vi "Unmarshal.vi"(8 "error in (no error)":errorcluster, 10 "Buffer":u8[](array[numeric]), 11 "int32 in":refnum<class "double.lvclass">) -> (0 "error out":errorcluster, 2 "Buffer Count":i32=8, 3 "int32 out":refnum<class "double.lvclass">)   [LabVIEW 2020, in "Protobuf RAW.lvlib" / "double.lvclass"]
uses:
  double.lvclass
  double.lvclass/double.ctl
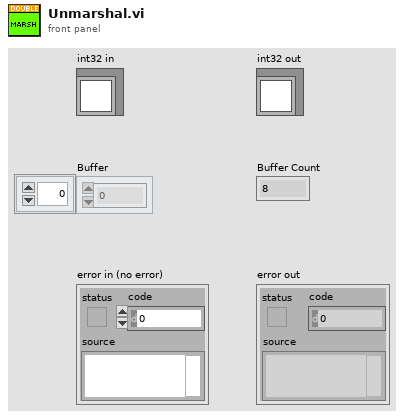
[diagram p1: front panel]
types:
  T1 = enum16{"big-endian, network order", "native, host order", "little-endian"}
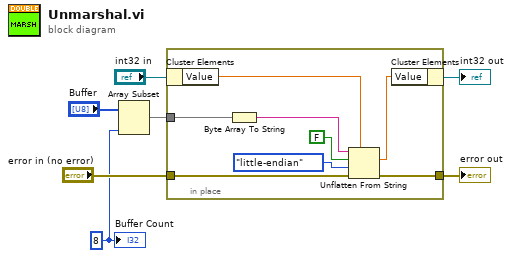
[diagram p0: block diagram]
diagram:
  w1 = 8 ("Buffer Count")
  n1 = Array Subset(array="Buffer", length=w1) -> (w2:u8[])  [unwired: 1 in]
  n2 = in-place {
    in-place-border: "error in (no error)" -> [w15]
    in-place-border: [w14] -> w4
    in-place-border: w2 -> [w9]
    n3 = in-place-cluster #1("int32 in") -> ("Value"=w13:dbl)
    n4 = Byte Array To String(unsigned byte array=w9) -> (string=w8:string)
    n5 = Unflatten From String(type=w13, binary string=w8, data includes array or string size? (T)=FALSE, byte order (0:big-endian, network order)=T1."little-endian", error in (no error)=w15) -> (value=w12:dbl, error out=w14:errorcluster)  [unwired: 1 out]
    n6 = in-place-cluster #1("Value"=w12) -> (→"int32 out":refnum<class "double.lvclass">)
  }
  "error out" <- w4
  "Buffer Count" <- w1
